vi "Main.vi"() -> ()   [LabVIEW 2026]
uses:
  statemachine.ctl
  <vilib>/numeric/Random Number (Range) DBL.vi
panel:
  out "em led":bool
  out "ready led":bool
  out "pause led":bool
  out "init led":bool
  out "run led":bool
  out "State":T1
  in  "Products":u16=50
  in  "speed":i32(listbox)
  out "need product":bool=TRUE
  in  "EMERGENCY":bool
  out "Thermometer":dbl(slide)=22.025379166725855 scale=0.0..200.0
  in  "RPM x1000":dbl(knob)=-1.0296070099394212 scale=0.0..10.0
  in  "STOP":bool
  in  "Machine Start":bool
  in  "PAUSE":bool
  # "CONTROLS"
  # "MACHINE PARAMETERS"
  # "SPEED"
  # "PRODUCT"
  # "STATE"
  # "TEMPERATURE"
  # "RPM x1000"
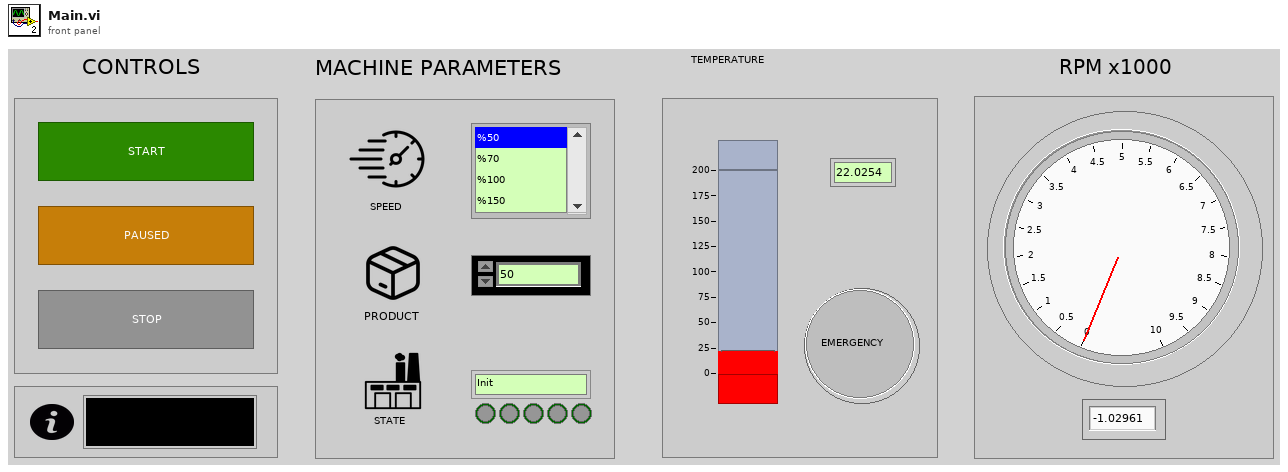
[diagram p1: front panel]
types:
  T1 = typedef "statemachine.ctl" = enum16{"Init", "Ready", "Running", "Paused", "Emergency"}
  T2 = cluster{"Products":u16, "RPM x1000":dbl, "speed":i32, "Thermometer":dbl, "EMERGENCY":bool}
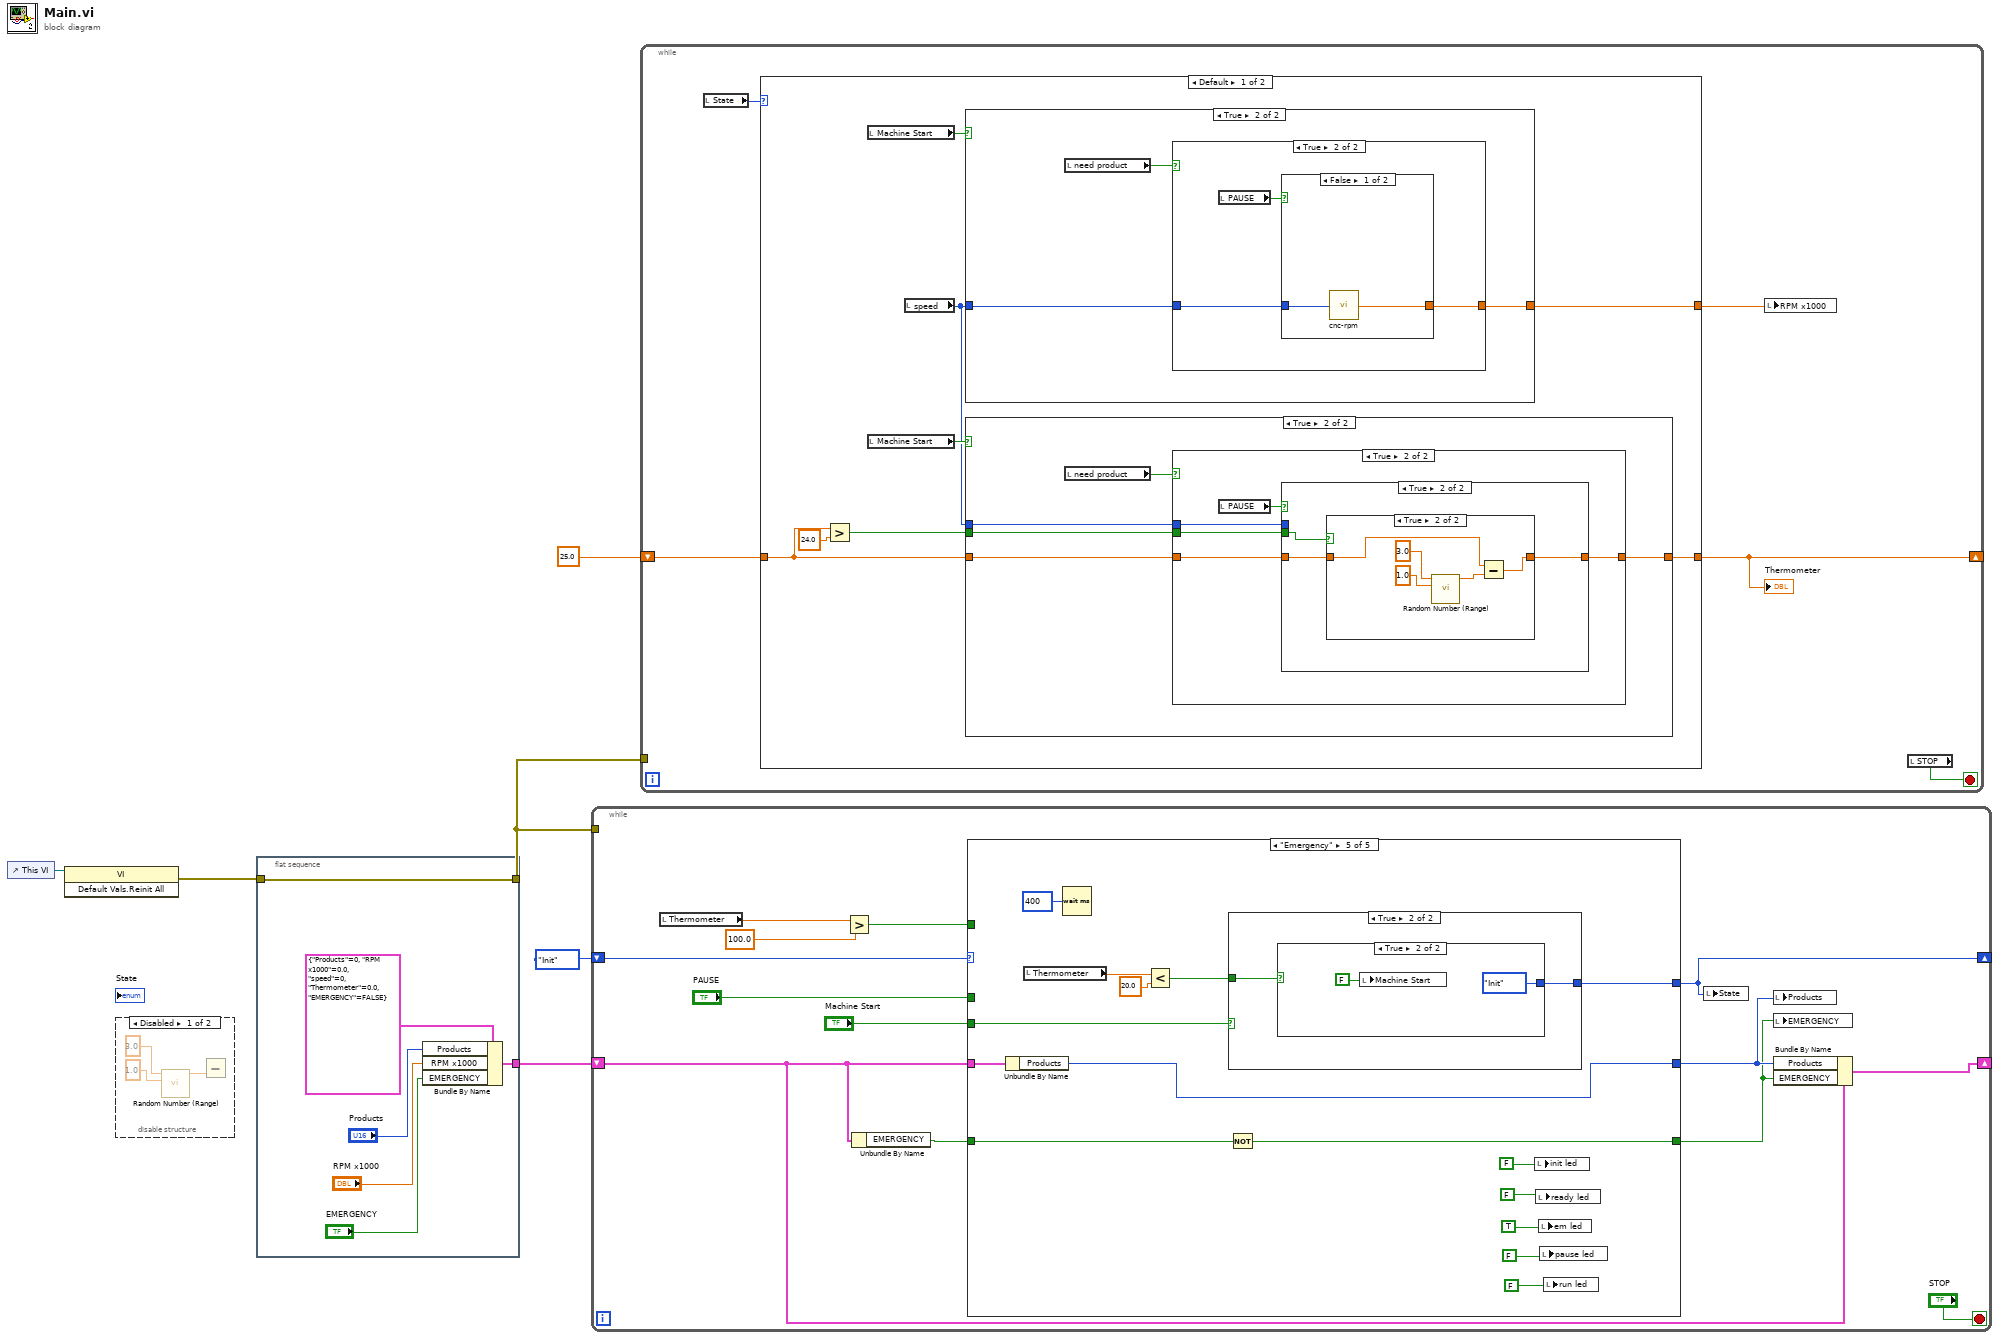
[diagram p0: block diagram]
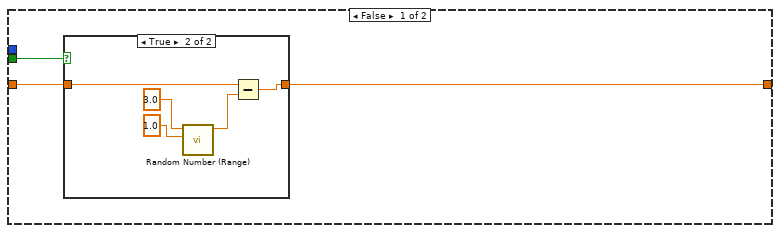
[diagram p3: hidden frame]
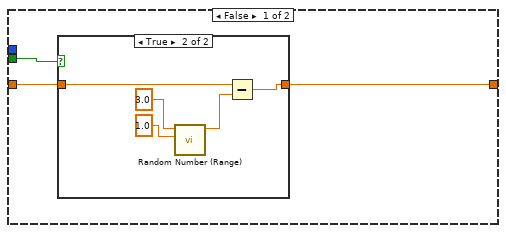
[diagram p5: hidden frame]
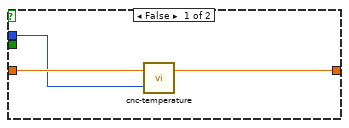
[diagram p7: hidden frame]
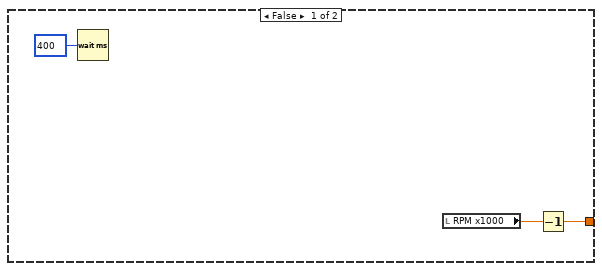
[diagram p9: hidden frame]
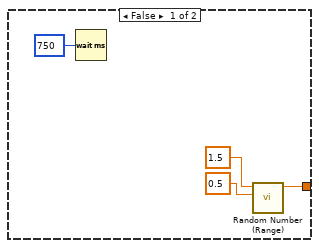
[diagram p10: hidden frame]
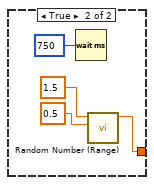
[diagram p11: hidden frame]
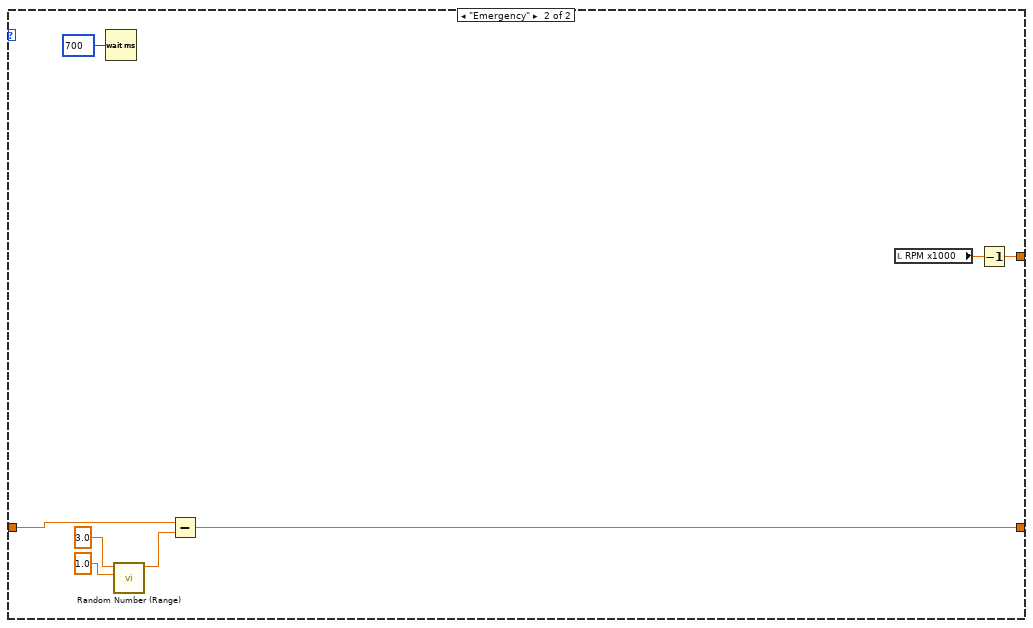
[diagram p12: hidden frame]
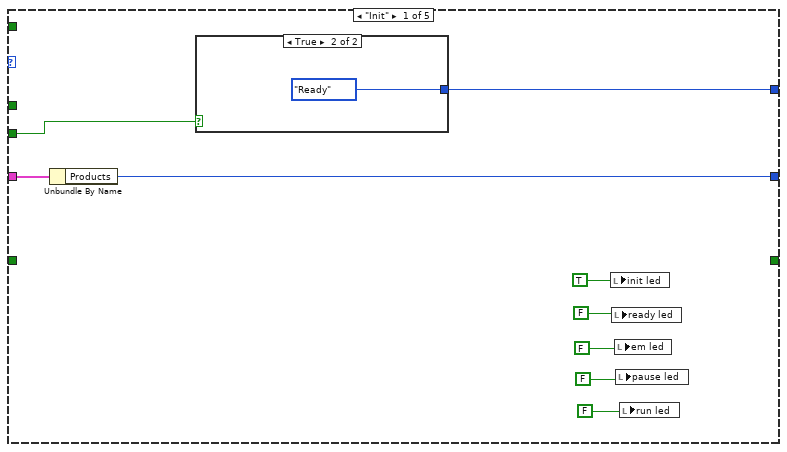
[diagram p13: hidden frame]
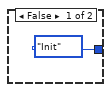
[diagram p14: hidden frame]
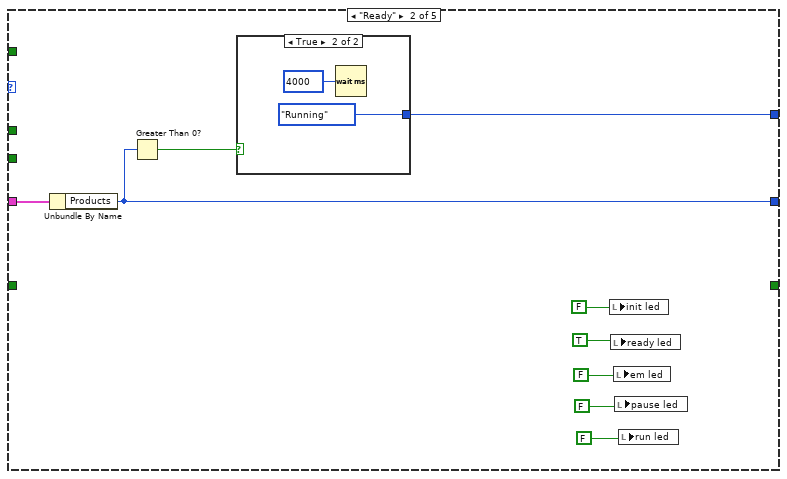
[diagram p15: hidden frame]
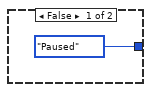
[diagram p16: hidden frame]
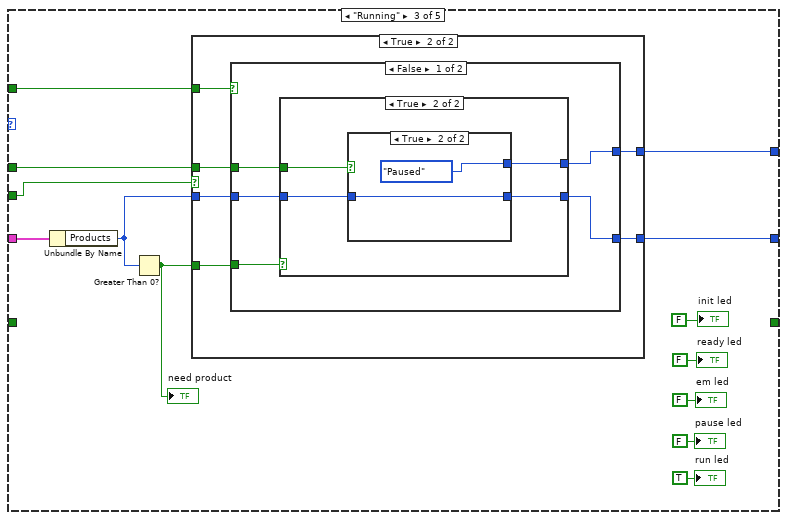
[diagram p17: hidden frame]
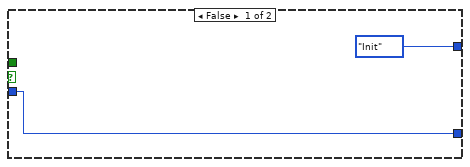
[diagram p18: hidden frame]
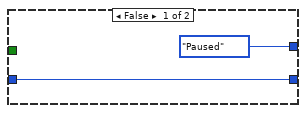
[diagram p19: hidden frame]
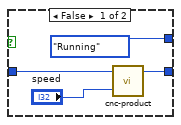
[diagram p20: hidden frame]
diagram:
  n1 = control-ref of="This VI"() -> (w3:refnum<vi>)
  n2 = invoke class="VI" method="Default Vals.Reinit All"(reference=w3) -> (error out=w2:errorcluster)  [unwired: 2 in, 2 out]
  n3 = disable-structure shown="Disabled" {
    frame Disabled {
      n4 = call-poly <vilib>:"Random Number (Range).vi"("lower bound (0)"=1.0, "upper bound (100)"=3.0) -> ("number"=w10:dbl)  [unwired: 9 in]
      n5 = Subtract(y=w10) -> (x=w9:dbl)  [unwired: 1 out]
    }
    frame Enabled {
    }
  }
  n6 = flat-sequence {
    tunnel: [w16] -> w6
    tunnel: w2 -> [w11]
    tunnel: [w11] -> w1
    frame #0 {
      n7 = Bundle By Name(cluster=T2 {"Products"=0, "RPM x1000"=0.0, "speed"=0, "Thermometer"=0.0, "EMERGENCY"=FALSE}, "Products"="Products", "RPM x1000"="RPM x1000", "EMERGENCY"="EMERGENCY") -> (w16:T2)
    }
  }
  n8 = while {
    shift-right: [w27] -> _
    shift-left: statemachine."Init" ("Enum") -> [w28]
    shift-right: [w26] -> _
    shift-left: w6 -> [w21]
    tunnel: w1 -> [_]
    stop <- "STOP" stop-if-true
    n9 = local read "Thermometer"() -> (w22:dbl)
    n10 = Greater?(x=w22, y=100.0) -> (0:w23:bool)
    n11 = Unbundle By Name(w21) -> ("EMERGENCY"=w19:bool)
    n12 = case shown="\"Emergency\"" w28 {
      tunnel: [w36 w49 w65 w102 w120] -> w27
      tunnel: [w38 w47 w64 w104 w121] -> w25
      tunnel: "Machine Start" -> [w37 _ w53 _ w112]
      tunnel: "PAUSE" -> [_ _ w59 w103 _]
      tunnel: w21 -> [w35 w46 w63 w100 w119]
      tunnel: w23 -> [_ _ w61 _ _]
      tunnel: [_ _ _ _ w115] -> w20
      tunnel: w19 -> [_ _ _ _ w116]
      frame "Init" {
        n13 = Unbundle By Name(w35) -> ("Products"=w38:u16)
        n14 = case shown="True" w37 {
          tunnel: [statemachine."Init" ("Enum") statemachine."Ready" ("Enum")] -> w36
          frame False {
          }
          frame True {
          }
        }
        n15 = local write "init led"(TRUE) -> ()
        n16 = local write "ready led"(FALSE) -> ()
        n17 = local write "em led"(FALSE) -> ()
        n18 = local write "pause led"(FALSE) -> ()
        n19 = local write "run led"(FALSE) -> ()
      }
      frame "Ready" {
        n20 = Unbundle By Name(w46) -> ("Products"=w47:u16)
        n21 = Greater Than 0?(x=w47) -> (x > 0?=w48:bool)
        n22 = case shown="True" w48 {
          tunnel: [statemachine."Paused" ("Enum") statemachine."Running" ("Enum")] -> w49
          frame False {
          }
          frame True {
            n23 = Wait (ms)(milliseconds to wait=u32 4000) -> ()  [unwired: 1 out]
          }
        }
        n24 = local write "init led"(FALSE) -> ()
        n25 = local write "ready led"(TRUE) -> ()
        n26 = local write "em led"(FALSE) -> ()
        n27 = local write "pause led"(FALSE) -> ()
        n28 = local write "run led"(FALSE) -> ()
      }
      frame "Running" {
        n29 = Unbundle By Name(w63) -> ("Products"=w62:u16)
        n30 = Greater Than 0?(x=w62) -> (x > 0?=w60:bool)
        "need product" <- w60
        n31 = case shown="True" w53 {
          tunnel: [statemachine."Init" ("Enum") w73] -> w65
          tunnel: [w66 w72] -> w64
          tunnel: w62 -> [w66 w71]
          tunnel: w61 -> [_ w70]
          tunnel: w60 -> [_ w69]
          tunnel: w59 -> [_ w68]
          frame False {
          }
          frame True {
            n32 = case shown="False" w70 {
              tunnel: [w77 statemachine."Emergency" ("Enum")] -> w73
              tunnel: [w78 w93] -> w72
              tunnel: w71 -> [w76 w93]
              tunnel: w69 -> [w75 _]
              tunnel: w68 -> [w74 _]
              frame False {
                n33 = case shown="True" w75 {
                  tunnel: [w80 w84] -> w78
                  tunnel: [statemachine."Paused" ("Enum") w83] -> w77
                  tunnel: w76 -> [w80 w82]
                  tunnel: w74 -> [_ w81]
                  frame False {
                  }
                  frame True {
                    n34 = case shown="True" w81 {
                      tunnel: [w88 w90] -> w84
                      tunnel: [statemachine."Running" ("Enum") statemachine."Paused" ("Enum")] -> w83
                      tunnel: w82 -> [w86 w90]
                      frame False {
                        n35 = call "cnc-product.vi"("speed in"="speed", "Products in"=w86) -> ("Products out"=w88:u16)  [unwired: 1 in]
                      }
                      frame True {
                      }
                    }
                  }
                }
              }
              frame True {
                n36 = local write "EMERGENCY"(TRUE ("EMERGENCY")) -> ()
                n37 = Wait (ms)(milliseconds to wait=u32 400) -> ()  [unwired: 1 out]
              }
            }
          }
        }
        "em led" <- FALSE
        "pause led" <- FALSE
        "ready led" <- FALSE
        "init led" <- FALSE
        "run led" <- TRUE
      }
      frame "Paused" {
        n38 = Unbundle By Name(w100) -> ("Products"=w104:u16)
        n39 = Wait (ms)(milliseconds to wait=u32 750) -> ()  [unwired: 1 out]
        n40 = case shown="False" w103 {
          tunnel: [statemachine."Running" ("Enum") statemachine."Paused" ("Enum")] -> w102
          frame False {
          }
          frame True {
          }
        }
        n41 = local write "init led"(FALSE) -> ()
        n42 = local write "ready led"(FALSE) -> ()
        n43 = local write "em led"(FALSE) -> ()
        n44 = local write "pause led"(TRUE) -> ()
        n45 = local write "run led"(FALSE) -> ()
      }
      frame "Emergency" {
        n46 = Unbundle By Name(w119) -> ("Products"=w121:u16)
        n47 = local read "Thermometer"() -> (w118:dbl)
        n48 = Wait (ms)(milliseconds to wait=u32 400) -> ()  [unwired: 1 out]
        n49 = Less?(x=w118, y=20.0) -> (x < y?=w113:bool)
        n50 = case shown="True" w112 {
          tunnel: [statemachine."Emergency" ("Enum") w124] -> w120
          tunnel: w113 -> [_ w123]
          frame False {
          }
          frame True {
            n51 = case shown="True" w123 {
              tunnel: [statemachine."Emergency" ("Enum") statemachine."Init" ("Enum")] -> w124
              frame False {
              }
              frame True {
                n52 = local write "Machine Start"(FALSE) -> ()
              }
            }
          }
        }
        n53 = Not(x=w116) -> (.not. x?=w115:bool)
        n54 = local write "init led"(FALSE) -> ()
        n55 = local write "ready led"(FALSE) -> ()
        n56 = local write "em led"(TRUE) -> ()
        n57 = local write "pause led"(FALSE) -> ()
        n58 = local write "run led"(FALSE) -> ()
      }
    }
    n59 = local write "State"(w27) -> ()
    n60 = local write "Products"(w25) -> ()
    n61 = local write "EMERGENCY"(w20) -> ()
    n62 = Bundle By Name(cluster=w21, "Products"=w25, "EMERGENCY"=w20) -> (w26:T2)
  }
  n63 = while {
    shift-right: [w130] -> _
    shift-left: 25.0 ("Thermometer") -> [w131]
    tunnel: w1 -> [_]
    stop <- w132 stop-if-true
    n64 = local read "State"() -> (w128:T1)
    n65 = case shown="Default" w128 {
      tunnel: w131 -> [w134 w204]
      tunnel: [w137 w203] -> w130
      tunnel: [w133 w200] -> w129
      frame Default {
        n66 = Greater?(x=w134, y=24.0 ("Thermometer")) -> (0:w135:bool)
        n67 = local read "Machine Start"() -> (w140:bool)
        n68 = local read "Machine Start"() -> (w139:bool)
        n69 = local read "speed"() -> (w138:i32)
        n70 = case shown="True" w140 {
          tunnel: w138 -> [_ w186]
          tunnel: [w182 w185] -> w133
          frame False {
            n71 = Wait (ms)(milliseconds to wait=u32 400) -> ()  [unwired: 1 out]
            n72 = local read "RPM x1000"() -> (w183:dbl)
            n73 = Decrement(x=w183) -> (x-1=w182:dbl)
          }
          frame True {
            n74 = local read "need product"() -> (w184:bool)
            n75 = case shown="True" w184 {
              tunnel: w186 -> [_ w192]
              tunnel: [w187 w191] -> w185
              frame False {
                n76 = Wait (ms)(milliseconds to wait=u32 750) -> ()  [unwired: 1 out]
                n77 = call-poly <vilib>:"Random Number (Range).vi"("lower bound (0)"=0.5, "upper bound (100)"=1.5) -> ("number"=w187:dbl)  [unwired: 9 in]
              }
              frame True {
                n78 = local read "PAUSE"() -> (w193:bool)
                n79 = case shown="False" w193 {
                  tunnel: w192 -> [w195 _]
                  tunnel: [w194 w197] -> w191
                  frame False {
                    n80 = call "cnc-rpm.vi"("speed in"=w195) -> ("rpm out"=w194:dbl)
                  }
                  frame True {
                    n81 = Wait (ms)(milliseconds to wait=u32 750) -> ()  [unwired: 1 out]
                    n82 = call-poly <vilib>:"Random Number (Range).vi"("lower bound (0)"=0.5, "upper bound (100)"=1.5) -> ("number"=w197:dbl)  [unwired: 9 in]
                  }
                }
              }
            }
          }
        }
        n83 = case shown="True" w139 {
          tunnel: w134 -> [w143 w153]
          tunnel: w138 -> [_ w152]
          tunnel: [w142 w151] -> w137
          tunnel: w135 -> [w141 w150]
          frame False {
            n84 = case shown="True" w141 {
              tunnel: w143 -> [w144 w146]
              tunnel: [w144 w145] -> w142
              frame False {
              }
              frame True {
                n85 = call-poly <vilib>:"Random Number (Range).vi"("lower bound (0)"=1.0, "upper bound (100)"=3.0) -> ("number"=w149:dbl)  [unwired: 9 in]
                n86 = Subtract(x=w146, y=w149) -> (x-y=w145:dbl)
              }
            }
          }
          frame True {
            n87 = local read "need product"() -> (w154:bool)
            n88 = case shown="True" w154 {
              tunnel: w153 -> [w156 w167]
              tunnel: w152 -> [_ w166]
              tunnel: [w157 w165] -> w151
              tunnel: w150 -> [w155 w164]
              frame False {
                n89 = case shown="True" w155 {
                  tunnel: [w158 w160] -> w157
                  tunnel: w156 -> [w158 w159]
                  frame False {
                  }
                  frame True {
                    n90 = call-poly <vilib>:"Random Number (Range).vi"("lower bound (0)"=1.0, "upper bound (100)"=3.0) -> ("number"=w163:dbl)  [unwired: 9 in]
                    n91 = Subtract(x=w159, y=w163) -> (x-y=w160:dbl)
                  }
                }
              }
              frame True {
                n92 = local read "PAUSE"() -> (w168:bool)
                n93 = case shown="True" w168 {
                  tunnel: w167 -> [w171 w174]
                  tunnel: w166 -> [w170 _]
                  tunnel: [w169 w173] -> w165
                  tunnel: w164 -> [_ w172]
                  frame False {
                    n94 = call "cnc-temperature.vi"("speed in"=w170, "Temperature in"=w171) -> ("Temperature out"=w169:dbl)  [unwired: 1 in]
                  }
                  frame True {
                    n95 = case shown="True" w172 {
                      tunnel: w174 -> [w175 w177]
                      tunnel: [w175 w176] -> w173
                      frame False {
                      }
                      frame True {
                        n96 = call-poly <vilib>:"Random Number (Range).vi"("lower bound (0)"=1.0, "upper bound (100)"=3.0) -> ("number"=w178:dbl)  [unwired: 9 in]
                        n97 = Subtract(x=w177, y=w178) -> (x-y=w176:dbl)
                      }
                    }
                  }
                }
              }
            }
          }
        }
      }
      frame "Emergency" {
        n98 = Wait (ms)(milliseconds to wait=u32 700) -> ()  [unwired: 1 out]
        n99 = call-poly <vilib>:"Random Number (Range).vi"("lower bound (0)"=1.0, "upper bound (100)"=3.0) -> ("number"=w207:dbl)  [unwired: 9 in]
        n100 = Subtract(x=w204, y=w207) -> (x-y=w203:dbl)
        n101 = local read "RPM x1000"() -> (w202:dbl)
        n102 = Decrement(x=w202) -> (x-1=w200:dbl)
      }
    }
    "Thermometer" <- w130
    n103 = local write "RPM x1000"(w129) -> ()
    n104 = local read "STOP"() -> (w132:bool)
  }
